vi "Get ODs from Buffer.vi"(8 "error in (no error)":errorcluster, 11 "Data":refnum<vi>) -> (0 "error out":errorcluster, 3 "data":T1[](array[typedef]) {"SubNumber" format="%x"; "AccessType" items=["", "ro", "wo", "rw", "const", "rwr", "rww"]; "DataType" items=[""=0, "BOOLEAN"=1, "INTEGER8"=2, "INTEGER16"=3, "INTEGER32"=4, "UNSIGNED8"=5, "UNSIGNED16"=6, "UNSIGNED32"=7, "REAL32"=8, "VISIBLE_STRING"=9, "OCTET_STRING"=10, "UNICODE_STRING"=11, "TIME_OF_DAY"=12, "TIME_DIFFERENCE"=13, "DOMAIN"=15, "INTEGER24"=16, "REAL64"=17, "INTEGER40"=18, "INTEGER48"=19, "INTEGER56"=20, "INTEGER64"=21, "UNSIGNED24"=22, "UNSIGNED40"=24, "UNSIGNED48"=25, "UNSIGNED56"=26, "UNSIGNED64"=27]; "ObjectType" items=[""=10, "NULL"=0, "DOMAIN"=2, "DEFTYPE"=5, "DEFSTRUCT"=6, "VAR"=7, "ARRAY"=8, "RECORD"=9]; "sub-index" format="%x"; "index" format="%x"})   [LabVIEW 2013]
uses:
  control/OD Entry.ctl
  control/Object Type.ctl
  control/Data Type.ctl
  control/Access Type.ctl
  control/OD Cateory.ctl
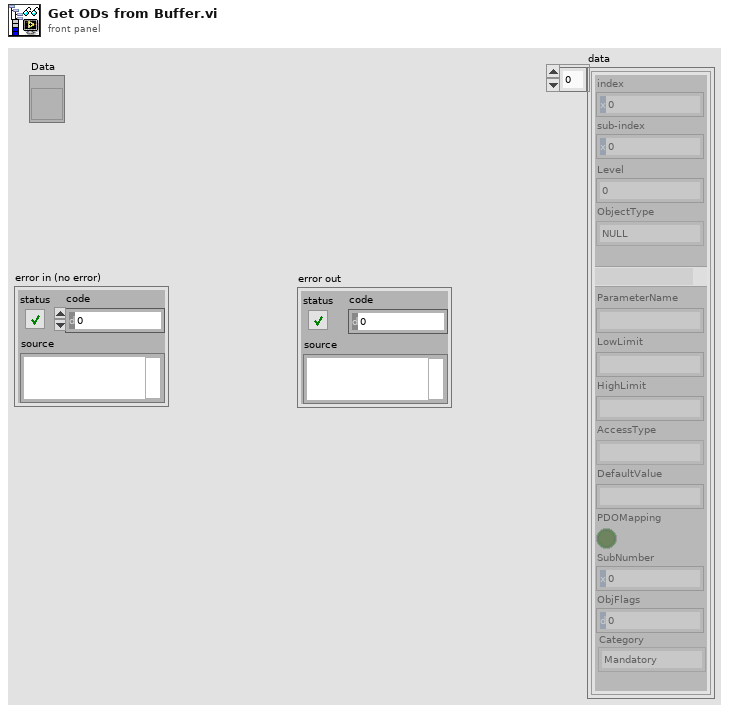
[diagram p1: front panel]
types:
  T1 = typedef "OD Entry.ctl" = cluster{"index":u16, "sub-index":u8, "Level":u8, "ObjectType":T2, "DataType":T3, "ParameterName":string, "LowLimit":string, "HighLimit":string, "AccessType":T4, "DefaultValue":string, "PDOMapping":bool, "SubNumber":u8, "ObjFlags":u32, "Category":T5}
  T2 = typedef "Object Type.ctl" = u16
  T3 = typedef "Data Type.ctl" = u16
  T4 = typedef "Access Type.ctl" = u16
  T5 = typedef "OD Cateory.ctl" = enum16{"Mandatory", "Optional", "Manufacturer", ""}
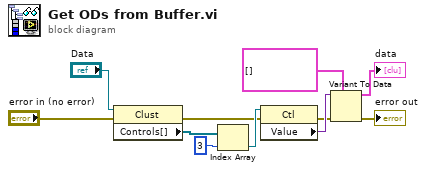
[diagram p0: block diagram]
diagram:
  n1 = property class="Clust"(reference="Data", error in="error in (no error)") -> (error out=w7:errorcluster, "Controls[]"=w10:refnum<vi>[])  [unwired: 1 out]
  n2 = Index Array(array=w10, index=3) -> (element=w8:refnum<vi>)
  n3 = property class="Ctl"(reference=w8, error in=w7) -> (error out=w5:errorcluster, "Value"=w6:variant)  [unwired: 1 out]
  n4 = Variant To Data(error in=w5, type=T1[] [], Variant=w6) -> (data=→"data":T1[], error out=→"error out":errorcluster)
